vi "set_triggered.vi"(8 "error in (no error)":errorcluster, 10 "triggered?":bool, 11 "FPGAWrapperDL090211Galvo in":refnum<class "FPGAWrapperMM140723Galvo.lvclass">) -> (0 "error out":errorcluster, 3 "FPGAWrapperDL090211Galvo out":refnum<class "FPGAWrapperMM140723Galvo.lvclass">)   [LabVIEW 2010, in "FPGAWrapperMM140723Galvo.lvclass"]
uses:
  FPGAWrapperMM140723Galvo.lvclass
  FPGAWrapperMM140723Galvo.lvclass/FPGAWrapperMM140723Galvo.ctl
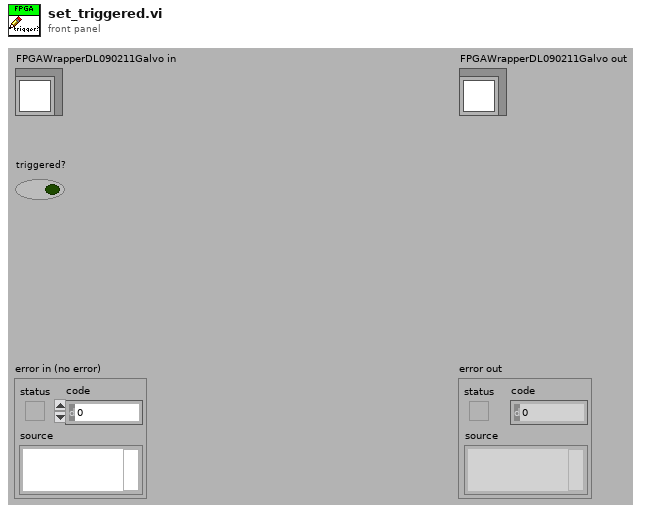
[diagram p1: front panel]
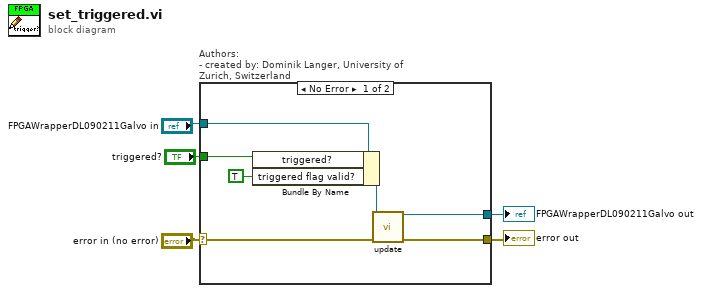
[diagram p0: block diagram]
diagram:
  n1 = case "Authors: \n- created by: Dominik Langer, University of Zurich, Switzerland" shown="No Error" "error in (no error)" {
    selector: "error in (no error)" -> [w10 w13]
    tunnel: "FPGAWrapperDL090211Galvo in" -> [w11 w14]
    tunnel: [w8 w14] -> w4
    tunnel: [w9 w13] -> w5
    tunnel: "triggered?" -> [w12 _]
    frame No Error {
      n2 = Bundle By Name(cluster=w11, "triggered?"=w12, "triggered flag valid?"=TRUE ("settings.triggered flag valid?")) -> (w7:refnum<class "FPGAWrapperMM140723Galvo.lvclass">)
      n3 = call-dynamic "update.vi"("error in (no error)"=w10, "FPGAWrapperDL120115Galvo in"=w7) -> ("error out"=w9:errorcluster, "FPGAWrapperDL120115Galvo out"=w8:refnum<class "FPGAWrapperMM140723Galvo.lvclass">)  [unwired: 8 in]
    }
    frame Error {
    }
  }
  "error out" <- w5
  "FPGAWrapperDL090211Galvo out" <- w4
